vi "CASCADE LED AND LOGO VALIDATION_PATTERN_MATCH.VI"(0 "Color Plane (Color Plane Extraction 1)":i32(ring)=1 items=["Red", "Green", "Blue", "Hue", "Saturation", "Luminance", "Value", "Intensity"], 1 "Template File Path (Pattern Locate Datum)":path=path "C:/mtp/Site_Ne_sch/Projects/DS4608_FAT/IMAGES/Datum_Right1.png", 2 "Template File Path (Pattern Match CENTER_LED)":path=path "C:/mtp/Site_Ne_sch/Projects/DS4608_FAT/IMAGES/Status LED.png", 3 "Template File Path (Pattern Matching LOGO)":path=path "C:/mtp/Site_Ne_sch/Projects/DS4608_FAT/IMAGES/Zebra_Logo.png", 7 "error in":errorcluster, 8 "Image File Path":path=path "C:/SNAPSHOT.bmp") -> (20 "Matches (Pattern Locate Datum)":T2(array[cluster]) {"Bounding Box"."y" format="%.2f"; "Bounding Box"."x" format="%.2f"; "Position"."y" format="%.2f"; "Position"."x" format="%.2f"; "Score" format="%.2f"; "Scale" format="%.2f"; "Angle" format="%.2f"}, 21 "Number of Matches (Pattern Locate Datum)":i32, 22 "Matches (Pattern Match CENTER_LED)":T2(array[cluster]) {"Bounding Box"."y" format="%.2f"; "Bounding Box"."x" format="%.2f"; "Position"."y" format="%.2f"; "Position"."x" format="%.2f"; "Score" format="%.2f"; "Scale" format="%.2f"; "Angle" format="%.2f"}, 23 "Number of Matches (Pattern Match CENTER_LED)":i32, 24 "Matches (Pattern Matching LOGO)":T2(array[cluster]) {"Bounding Box"."y" format="%.2f"; "Bounding Box"."x" format="%.2f"; "Position"."y" format="%.2f"; "Position"."x" format="%.2f"; "Score" format="%.2f"; "Scale" format="%.2f"; "Angle" format="%.2f"}, 25 "Number of Matches (Pattern Matching LOGO)":i32, 27 "error out":errorcluster)   [LabVIEW 2014]
uses:
  <vilib>/vision/NI_Vision_Development_Module.lvlib
panel:
  out "Image Out":T1(plugin-control)
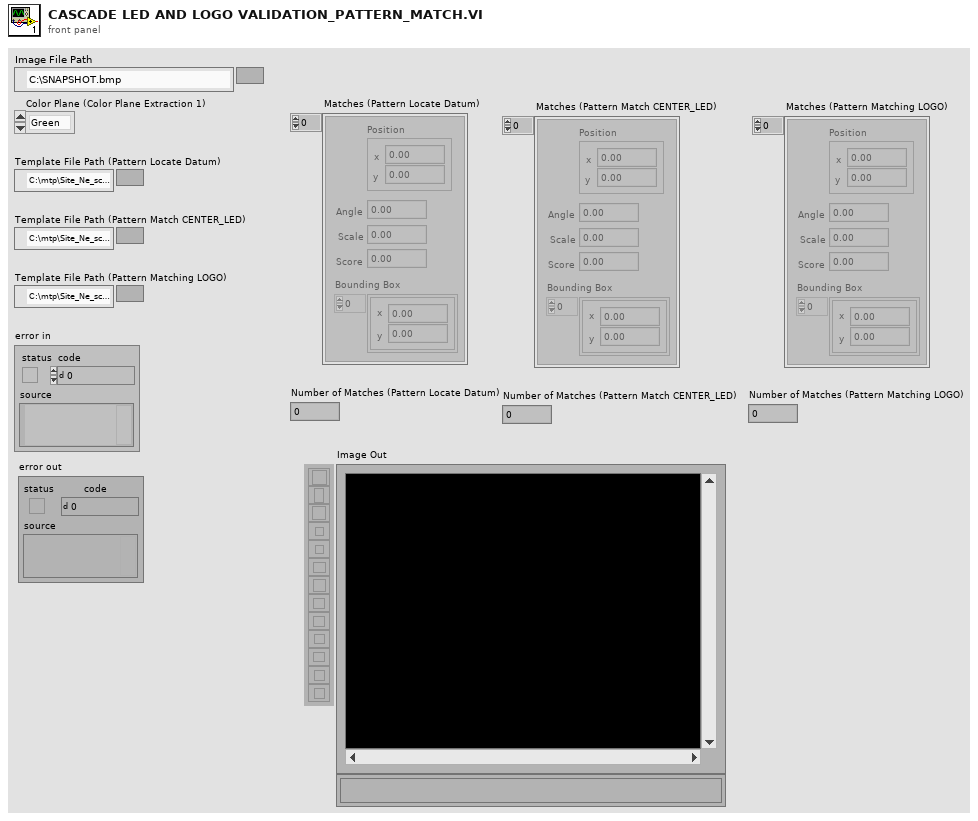
[diagram p1: front panel]
types:
  T1 = typedef "IMAQ Image.ctl" = refnum<image>
  T2 = cluster{"Position":cluster{"x":sgl, "y":sgl}, "Angle":sgl, "Scale":sgl, "Score":sgl, "Bounding Box":cluster{"x":sgl, "y":sgl}[]}[]
  T3 = cluster{"Number of Matches Requested":i32, "Minimum Match Score":sgl, "Angle Ranges":cluster{"Start Angle":sgl, "End Angle":sgl}[]}
  T4 = cluster{"Global Rectangle":i32[], "Contours":cluster{"ID":enum32{"External", "Internal"}, "Type":u32, "Coordinates":i32[]}[]}
  T5 = enum16{"Reset", "Update Coordinate System", "Get Coordinate System"}
  T6 = enum16{"Horizontal Motion", "Vertical Motion", "Horizontal and Vertical Motion", "Horizontal, Vertical and Angular Motion"}
  T7 = cluster{"Origin":cluster{"X":sgl, "Y":sgl}, "Angle (deg)":sgl, "Axis Reference":u32}
  T8 = typedef "Image Type" = u32
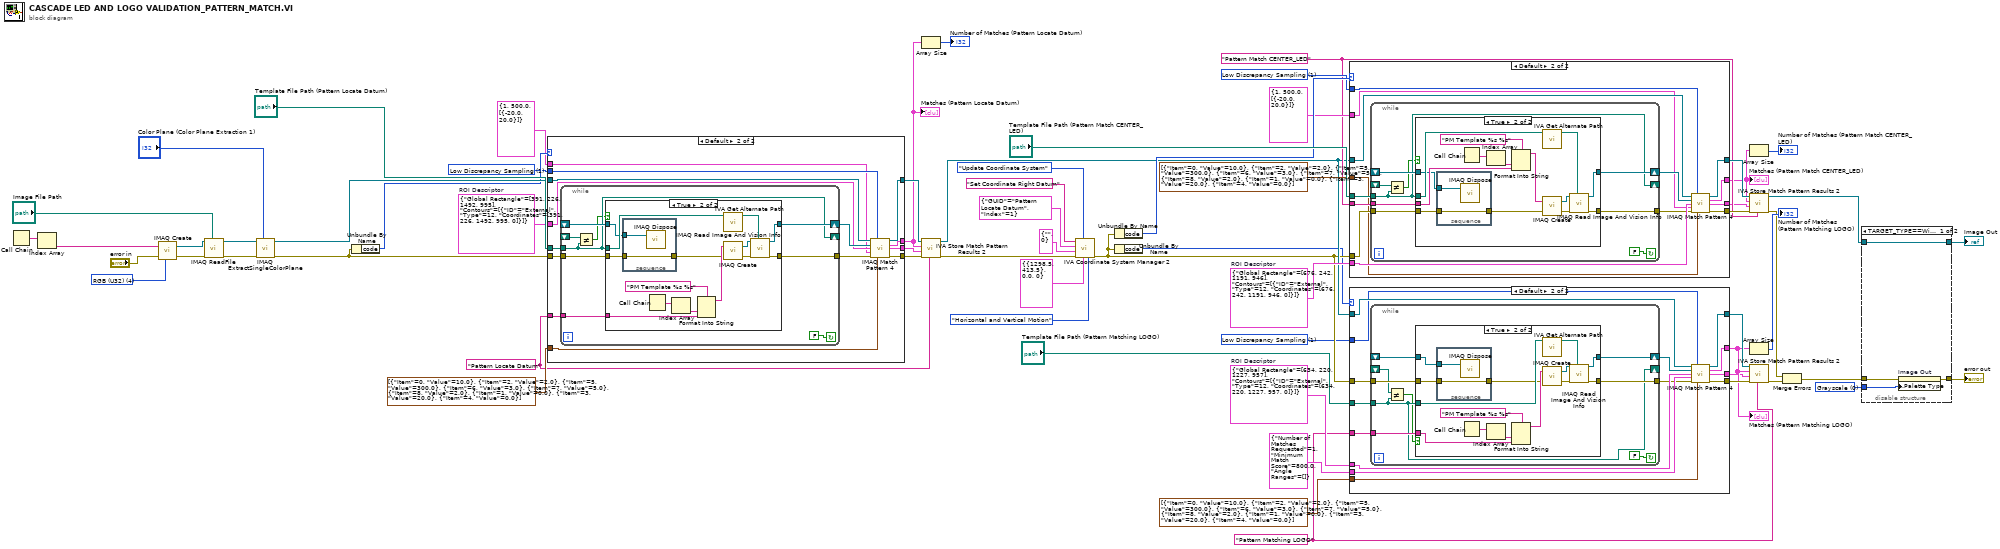
[diagram p0: block diagram]
diagram:
  w2 = u32 0 items=["Grayscale", "Binary", "Gradient", "Rainbow", "Temperature", "User Defined"] ("Palette")
  w16 = 1 items=["All", "Low Discrepancy Sampling", "Grayscale Value Pyramid", "Gradients Pyramid"] ("Algorithm")
  w11 = "Pattern Matching LOGO" ("Step Name")
  w15 = T4 {"Global Rectangle"=[634, 220, 1227, 957], "Contours"=[{"ID"=enum."External", "Type"=12, "Coordinates"=[634, 220, 1227, 957, 0]}]}  # ROI Descriptor
  w30 = 1 items=["All", "Low Discrepancy Sampling", "Grayscale Value Pyramid", "Gradients Pyramid"] ("Algorithm")
  w25 = "Pattern Match CENTER_LED" ("Step Name")
  w29 = T4 {"Global Rectangle"=[676, 242, 1191, 946], "Contours"=[{"ID"=enum."External", "Type"=12, "Coordinates"=[676, 242, 1191, 946, 0]}]}  # ROI Descriptor
  w49 = 1 items=["All", "Low Discrepancy Sampling", "Grayscale Value Pyramid", "Gradients Pyramid"] ("Algorithm")
  w44 = "Pattern Locate Datum" ("Step Name")
  w48 = T4 {"Global Rectangle"=[391, 226, 1492, 995], "Contours"=[{"ID"=enum."External", "Type"=12, "Coordinates"=[391, 226, 1492, 995, 0]}]}  # ROI Descriptor
  w59 = T8 4 items=["Grayscale (U8)", "Grayscale (I16)", "Grayscale (SGL)", "Complex (CSG)", "RGB (U32)", "HSL (U32)", "RGB (U64)", "Grayscale (U16)"] ("Image Type")
  n1 = Call Chain() -> (call chain=w61:string[])
  n2 = Index Array(array=w61) -> (element=w60:string)  [unwired: 1 in]
  n3 = call "IMAQ Create"("Image Name"=w60, "Image Type"=w59, "error in (no error)"="error in") -> ("New Image"=w64:T1, "error out"=w63:errorcluster)  [unwired: 1 in, 1 out]
  n4 = call "IMAQ ReadFile"("File Path"="Image File Path", "error in (no error)"=w63, "Image"=w64) -> ("error out"=w56:errorcluster, "Image Out"=w57:T1)  [unwired: 2 in, 5 out]
  n5 = call "IMAQ ExtractSingleColorPlane"("Color Plane"="Color Plane (Color Plane Extraction 1)", "error in (no error)"=w56, "Image Src"=w57) -> ("error out"=w51:errorcluster, "Image Dst Out"=w54:T1)  [unwired: 1 in, 6 out]
  n6 = Unbundle By Name(w51) -> ("code"=w50:i32)
  n7 = case shown="Default" w50 {
    tunnel: "Template File Path (Pattern Locate Datum)" -> [_ w79]
    tunnel: w51 -> [_ w78]
    tunnel: w54 -> [w65 w73]
    tunnel: [_ w74] -> w53
    tunnel: [_ w75] -> w43
    tunnel: [w65 w72] -> w52
    tunnel: w44 -> [_ w77]
    tunnel: w49 -> [_ w71]
    tunnel: w48 -> [_ w70]
    tunnel: T3 {"Number of Matches Requested"=1, "Minimum Match Score"=500.0, "Angle Ranges"=[{"Start Angle"=-20.0, "End Angle"=20.0}]} ("Parameters") -> [_ w69]
    tunnel: cluster{"Item":u16, "Value":dbl}[] [{"Item"=0, "Value"=10.0}, {"Item"=2, "Value"=2.0}, {"Item"=5, "Value"=300.0}, {"Item"=6, "Value"=3.0}, {"Item"=7, "Value"=5.0}, {"Item"=8, "Value"=2.0}, {"Item"=1, "Value"=0.0}, {"Item"=3, "Value"=20.0}, {"Item"=4, "Value"=0.0}] ("Advanced Options") -> [_ w67]
    tunnel: [_ w66] -> w42
    frame -1074396199, -1074396198 {
      # "Discard Coordinate System Error"
    }
    frame Default {
      n8 = while {
        shift-right: [w88] -> w76
        shift-left: _ -> [w87]
        tunnel: [w85] -> w68
        tunnel: w78 -> [w84]
        tunnel: w79 -> [w81]
        tunnel: w77 -> [w83]
        shift-right: [w81] -> _
        shift-left: _ -> [w82]
        stop <- FALSE continue-if-true
        n9 = Not Equal?(x=w82, y=w81) -> (x != y?=w80:bool)
        n10 = case shown="True" w80 {
          tunnel: [w90 w102] -> w88
          tunnel: w87 -> [w90 w93]
          tunnel: [w89 w99] -> w85
          tunnel: w84 -> [w89 w92]
          tunnel: w81 -> [_ w95]
          tunnel: w83 -> [_ w96]
          frame False {
          }
          frame True {
            n11 = stacked-sequence {
              tunnel: w93 -> [w106]
              tunnel: w92 -> [w105]
              tunnel: [w105] -> w91
              frame #0 {
                n12 = call "IMAQ Dispose"("Image"=w106) -> ()  [unwired: 2 in, 4 out]
              }
            }
            n13 = Call Chain() -> (call chain=w98:string[])
            n14 = Index Array(array=w98) -> (element=w97:string)  [unwired: 1 in]
            n15 = Format Into String(format string="PM Template %s %s" ("Image Name"), w97, w96) -> (resulting string=w104:string)  [unwired: 2 in, 1 out]
            n16 = call <vilib>:"IVA Get Alternate Path.vi"("Path In"=w95) -> ("Path Out"=w94:path)  [unwired: 10 out]
            n17 = call "IMAQ Create"("Image Name"=w104, "error in (no error)"=w91) -> ("New Image"=w101:T1, "error out"=w100:errorcluster)  [unwired: 2 in, 1 out]
            n18 = call "IMAQ Read Image And Vision Info"("File Path"=w94, "error in (no error)"=w100, "Image"=w101) -> ("error out"=w99:errorcluster, "Image Out"=w102:T1)  [unwired: 1 in, 6 out]
          }
        }
      }
      n19 = call "IMAQ Match Pattern 4"("Image"=w73, "Algorithm"=w71, "Template Image"=w76, "ROI Descriptor"=w70, "Parameters"=w69, "error in (no error)"=w68, "Advanced Options"=w67) -> ("Image (duplicate)"=w72:T1, "Matches (pixel)"=w75:T2, "Matches (real-world)"=w66:T2, "error out"=w74:errorcluster)  [unwired: 4 in, 1 out]
    }
  }
  "Matches (Pattern Locate Datum)" <- w43
  n20 = Array Size(array=w43) -> (size(s)=→"Number of Matches (Pattern Locate Datum)":i32)
  n21 = call <vilib>:"IVA Store Match Pattern Results 2.vi"("Step Name"=w44, "error in (no error)"=w53, "Matches (real-world)"=w42, "Matches (pixel)"=w43, "Image in"=w52) -> ("error out"=w35:errorcluster, "Image dup"=w21:T1)  [unwired: 1 in, 4 out]
  n22 = call <vilib>:"IVA Coordinate System Manager 2.vi"("Mode"=T6."Horizontal and Vertical Motion", "Reference System"=T7 {"Origin"={"X"=1298.5, "Y"=413.5}, "Angle (deg)"=0.0, "Axis Reference"=0}, "Function"=T5."Update Coordinate System", "error in (no error)"=w35, "Angle ID"=cluster{"GUID":string, "Index":i32} {"GUID"="", "Index"=0}, "Origin ID"=cluster{"GUID":string, "Index":i32} {"GUID"="Pattern Locate Datum", "Index"=1}, "Coordinate System Name"="Set Coordinate Right Datum") -> ("error out"=w18:errorcluster)  [unwired: 4 out]
  n23 = Unbundle By Name(w18) -> ("code"=w31:i32)
  n24 = Unbundle By Name(w18) -> ("code"=w17:i32)
  n25 = case shown="Default" w31 {
    tunnel: "Template File Path (Pattern Match CENTER_LED)" -> [_ w121]
    tunnel: w18 -> [_ w120]
    tunnel: w21 -> [w107 w115]
    tunnel: [_ w116] -> w33
    tunnel: [_ w117] -> w24
    tunnel: [w107 w114] -> w32
    tunnel: w25 -> [_ w119]
    tunnel: w30 -> [_ w113]
    tunnel: w29 -> [_ w112]
    tunnel: T3 {"Number of Matches Requested"=1, "Minimum Match Score"=500.0, "Angle Ranges"=[{"Start Angle"=-20.0, "End Angle"=20.0}]} ("Parameters") -> [_ w111]
    tunnel: cluster{"Item":u16, "Value":dbl}[] [{"Item"=0, "Value"=10.0}, {"Item"=2, "Value"=2.0}, {"Item"=5, "Value"=300.0}, {"Item"=6, "Value"=3.0}, {"Item"=7, "Value"=5.0}, {"Item"=8, "Value"=2.0}, {"Item"=1, "Value"=0.0}, {"Item"=3, "Value"=20.0}, {"Item"=4, "Value"=0.0}] ("Advanced Options") -> [_ w109]
    tunnel: [_ w108] -> w23
    frame -1074396199, -1074396198 {
      # "Discard Coordinate System Error"
    }
    frame Default {
      n26 = while {
        shift-right: [w130] -> w118
        shift-left: _ -> [w129]
        tunnel: [w127] -> w110
        tunnel: w120 -> [w126]
        tunnel: w121 -> [w123]
        tunnel: w119 -> [w125]
        shift-right: [w123] -> _
        shift-left: _ -> [w124]
        stop <- FALSE continue-if-true
        n27 = Not Equal?(x=w124, y=w123) -> (x != y?=w122:bool)
        n28 = case shown="True" w122 {
          tunnel: [w132 w144] -> w130
          tunnel: w129 -> [w132 w135]
          tunnel: [w131 w141] -> w127
          tunnel: w126 -> [w131 w134]
          tunnel: w123 -> [_ w137]
          tunnel: w125 -> [_ w138]
          frame False {
          }
          frame True {
            n29 = stacked-sequence {
              tunnel: w135 -> [w148]
              tunnel: w134 -> [w147]
              tunnel: [w147] -> w133
              frame #0 {
                n30 = call "IMAQ Dispose"("Image"=w148) -> ()  [unwired: 2 in, 4 out]
              }
            }
            n31 = Call Chain() -> (call chain=w140:string[])
            n32 = Index Array(array=w140) -> (element=w139:string)  [unwired: 1 in]
            n33 = Format Into String(format string="PM Template %s %s" ("Image Name"), w139, w138) -> (resulting string=w146:string)  [unwired: 2 in, 1 out]
            n34 = call <vilib>:"IVA Get Alternate Path.vi"("Path In"=w137) -> ("Path Out"=w136:path)  [unwired: 10 out]
            n35 = call "IMAQ Create"("Image Name"=w146, "error in (no error)"=w133) -> ("New Image"=w143:T1, "error out"=w142:errorcluster)  [unwired: 2 in, 1 out]
            n36 = call "IMAQ Read Image And Vision Info"("File Path"=w136, "error in (no error)"=w142, "Image"=w143) -> ("error out"=w141:errorcluster, "Image Out"=w144:T1)  [unwired: 1 in, 6 out]
          }
        }
      }
      n37 = call "IMAQ Match Pattern 4"("Image"=w115, "Algorithm"=w113, "Template Image"=w118, "ROI Descriptor"=w112, "Parameters"=w111, "error in (no error)"=w110, "Advanced Options"=w109) -> ("Image (duplicate)"=w114:T1, "Matches (pixel)"=w117:T2, "Matches (real-world)"=w108:T2, "error out"=w116:errorcluster)  [unwired: 4 in, 1 out]
    }
  }
  "Matches (Pattern Match CENTER_LED)" <- w24
  n38 = case shown="Default" w17 {
    tunnel: "Template File Path (Pattern Matching LOGO)" -> [_ w163]
    tunnel: w18 -> [_ w162]
    tunnel: w21 -> [w149 w157]
    tunnel: [_ w158] -> w20
    tunnel: [_ w159] -> w10
    tunnel: [w149 w156] -> w19
    tunnel: w11 -> [_ w161]
    tunnel: w16 -> [_ w155]
    tunnel: w15 -> [_ w154]
    tunnel: T3 {"Number of Matches Requested"=1, "Minimum Match Score"=800.0, "Angle Ranges"=[]} ("Parameters") -> [_ w153]
    tunnel: cluster{"Item":u16, "Value":dbl}[] [{"Item"=0, "Value"=10.0}, {"Item"=2, "Value"=2.0}, {"Item"=5, "Value"=300.0}, {"Item"=6, "Value"=3.0}, {"Item"=7, "Value"=5.0}, {"Item"=8, "Value"=2.0}, {"Item"=1, "Value"=0.0}, {"Item"=3, "Value"=20.0}, {"Item"=4, "Value"=0.0}] ("Advanced Options") -> [_ w151]
    tunnel: [_ w150] -> w9
    frame -1074396199, -1074396198 {
      # "Discard Coordinate System Error"
    }
    frame Default {
      n39 = while {
        shift-right: [w172] -> w160
        shift-left: _ -> [w171]
        tunnel: [w169] -> w152
        tunnel: w162 -> [w168]
        tunnel: w163 -> [w165]
        tunnel: w161 -> [w167]
        shift-right: [w165] -> _
        shift-left: _ -> [w166]
        stop <- FALSE continue-if-true
        n40 = Not Equal?(x=w166, y=w165) -> (x != y?=w164:bool)
        n41 = case shown="True" w164 {
          tunnel: [w174 w186] -> w172
          tunnel: w171 -> [w174 w177]
          tunnel: [w173 w183] -> w169
          tunnel: w168 -> [w173 w176]
          tunnel: w165 -> [_ w179]
          tunnel: w167 -> [_ w180]
          frame False {
          }
          frame True {
            n42 = stacked-sequence {
              tunnel: w177 -> [w190]
              tunnel: w176 -> [w189]
              tunnel: [w189] -> w175
              frame #0 {
                n43 = call "IMAQ Dispose"("Image"=w190) -> ()  [unwired: 2 in, 4 out]
              }
            }
            n44 = Call Chain() -> (call chain=w182:string[])
            n45 = Index Array(array=w182) -> (element=w181:string)  [unwired: 1 in]
            n46 = Format Into String(format string="PM Template %s %s" ("Image Name"), w181, w180) -> (resulting string=w188:string)  [unwired: 2 in, 1 out]
            n47 = call <vilib>:"IVA Get Alternate Path.vi"("Path In"=w179) -> ("Path Out"=w178:path)  [unwired: 10 out]
            n48 = call "IMAQ Create"("Image Name"=w188, "error in (no error)"=w175) -> ("New Image"=w185:T1, "error out"=w184:errorcluster)  [unwired: 2 in, 1 out]
            n49 = call "IMAQ Read Image And Vision Info"("File Path"=w178, "error in (no error)"=w184, "Image"=w185) -> ("error out"=w183:errorcluster, "Image Out"=w186:T1)  [unwired: 1 in, 6 out]
          }
        }
      }
      n50 = call "IMAQ Match Pattern 4"("Image"=w157, "Algorithm"=w155, "Template Image"=w160, "ROI Descriptor"=w154, "Parameters"=w153, "error in (no error)"=w152, "Advanced Options"=w151) -> ("Image (duplicate)"=w156:T1, "Matches (pixel)"=w159:T2, "Matches (real-world)"=w150:T2, "error out"=w158:errorcluster)  [unwired: 4 in, 1 out]
    }
  }
  "Matches (Pattern Matching LOGO)" <- w10
  n51 = Array Size(array=w24) -> (size(s)=→"Number of Matches (Pattern Match CENTER_LED)":i32)
  n52 = call <vilib>:"IVA Store Match Pattern Results 2.vi"("Step Name"=w25, "error in (no error)"=w33, "Matches (real-world)"=w23, "Matches (pixel)"=w24, "Image in"=w32) -> ("error out"=w8:errorcluster, "Image dup"=w4:T1)  [unwired: 1 in, 4 out]
  n53 = Array Size(array=w10) -> (size(s)=→"Number of Matches (Pattern Matching LOGO)":i32)
  n54 = call <vilib>:"IVA Store Match Pattern Results 2.vi"("Step Name"=w11, "error in (no error)"=w20, "Matches (real-world)"=w9, "Matches (pixel)"=w10, "Image in"=w19) -> ("error out"=w7:errorcluster)  [unwired: 1 in, 5 out]
  n55 = Merge Errors(w8, w7) -> (w6:errorcluster)
  n56 = disable-structure "Conditional Disable Structure" shown="TARGET_TYPE==Windows" {
    disable-tunnel: w6 -> [w194 w195]
    disable-tunnel: [w193 w195] -> w5
    disable-tunnel: w4 -> [w192 w196]
    disable-tunnel: [w192 w196] -> w3
    disable-tunnel: w2 -> [w191 _]
    frame condition #0 (active) {
      n57 = property on="Image Out" class="ImageControl"(error in=w194, "Palette:Palette Type"=w191) -> (error out=w193:errorcluster)  [unwired: 1 in, 1 out]
    }
    frame condition #1 {
    }
  }
  "error out" <- w5
  "Image Out" <- w3
